vi "Init GUI.vi"(0 "GUI in":refnum<class "GUI.lvclass">, 1 "ConfigInterface":refnum<class "ConfigInterface.lvclass">, 2 "SVW":refnum<class "SharedVariableWrapper.lvclass">, 11 "error in (no error)":errorcluster) -> (4 "GUI":refnum<class "GUI.lvclass">, 13 "SVW out":refnum<class "SharedVariableWrapper.lvclass">, 15 "error out":errorcluster)   [LabVIEW 2019, in "GUI.lvclass"]
uses:
  GUI.lvclass
  ConfigInterface_class/ConfigInterface.lvclass
  SV_Wrap/SharedVariableWrapper.lvclass
  CmdData.ctl
  Shered Data.ctl
  WindowsState.ctl
  GUI.lvclass/GUI.ctl
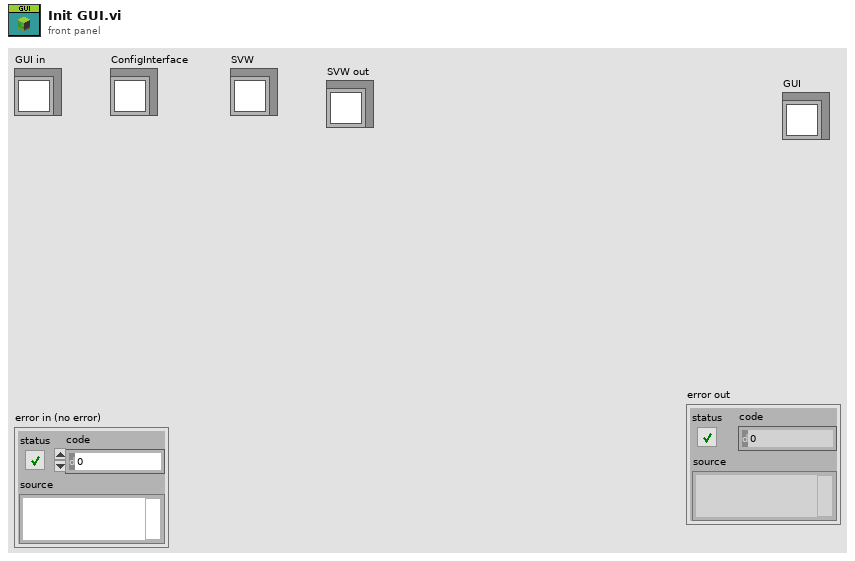
[diagram p1: front panel]
types:
  T1 = typedef "GUI.lvclass/CmdData.ctl" = cluster{"CMD":string, "DATA":variant}
  T2 = typedef "GUI.lvclass/Shered Data.ctl" = cluster{"WindowsState":T3, "UI VI":refnum<vi>, "SubPnl":refnum<vi>}
  T3 = typedef "GUI.lvclass/WindowsState.ctl" = enum16{"NotReady", "Ready", "Inserted", "Opened"}
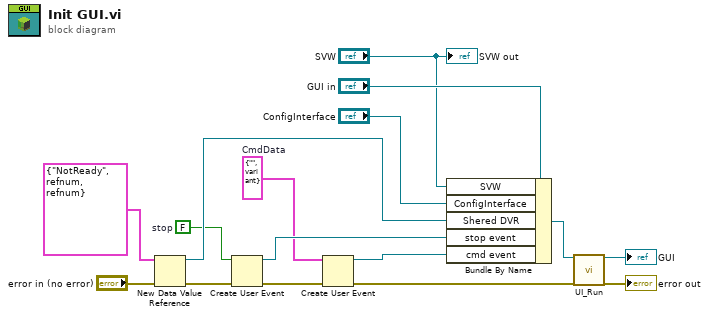
[diagram p0: block diagram]
diagram:
  w4 = T1 {"CMD"="", "DATA"=variant}  # CmdData
  w12 = FALSE  # stop
  n1 = New Data Value Reference(data value=T2 {"WindowsState"=enum."NotReady", "UI VI"=refnum, "SubPnl"=refnum} ("Shered Data"), error in="error in (no error)") -> (data value reference=w13:refnum<data-value>, error out=w11:errorcluster)
  n2 = Create User Event(user event datatype=w12, error in=w11) -> (user event=w10:refnum<user-event>, error out=w3:errorcluster)
  n3 = Create User Event(user event datatype=w4, error in=w3) -> (user event=w1:refnum<user-event>, error out=w2:errorcluster)
  n4 = Bundle By Name(cluster="GUI in", "SVW"="SVW", "ConfigInterface"="ConfigInterface", "Shered DVR"=w13, "stop event"=w10, "cmd event"=w1) -> (w9:refnum<class "GUI.lvclass">)
  n5 = call-dynamic "UI_Run.vi"("reference in"=w9, "error in (no error)"=w2) -> ("reference out"=→"GUI":refnum<class "GUI.lvclass">, "error out"=→"error out":errorcluster)  [unwired: 16 in]
  "SVW out" <- "SVW"
